vi "MecaKinematics_New.vi"(8 "RearRight":T1 {"Y" format="%14.3f"; "X" format="%14.3f"}, 9 "RearLeft":T1 {"Y" format="%14.3f"; "X" format="%14.3f"}, 10 "FrontRight":T1 {"Y" format="%14.3f"; "X" format="%14.3f"}, 11 "FrontLeft":T1 {"Y" format="%14.3f"; "X" format="%14.3f"}) -> (3 "MECA_DRIVE_KINEMATICS":T2={"FrontLeft"={"X"=0.0, "Y"=0.0}, "FrontRight"={"X"=0.0, "Y"=0.0}, "RearLeft"={"X"=0.0, "Y"=0.0}, "RearRight"={"X"=0.0, "Y"=0.0}, "InverseKinematics"=[[0.0, 1.0, -1.0, 0.0], [0.0, 1.0, 1.0, 0.0], [0.0, 1.0, 1.0, 0.0], [0.0, 1.0, -1.0, 0.0]], "ForwardKinematics"=[[0.0, 1.0, -1.0, 0.0], [0.0, 1.0, 1.0, 0.0], [0.0, 1.0, 1.0, 0.0], [0.0, 1.0, -1.0, 0.0]], "PrevCoR"={"X"=0.0, "Y"=0.0}} {"PrevCoR"."Y" format="%14.3f"; "PrevCoR"."X" format="%14.3f"; "RearRight"."Y" format="%14.3f"; "RearRight"."X" format="%14.3f"; "RearLeft"."Y" format="%14.3f"; "RearLeft"."X" format="%14.3f"; "FrontRight"."Y" format="%14.3f"; "FrontRight"."X" format="%14.3f"; "FrontLeft"."Y" format="%14.3f"; "FrontLeft"."X" format="%14.3f"})   [LabVIEW 2019, in "Trajectory_Library.lvlib"]
doc: "Constructs a MecanumDriveKinematics data structure.\n\nHelper class that converts a chassis velocity (dx, dy, and dtheta components) into individual wheel speeds.\n\nThe inverse kinematics (converting from a desired chassis velocity to individual wheel speeds) uses the relative locations of the wheels with respect to the center of rotation. The center of rotation for inverse kinematics is also variable. This means that you can set your set your center of rotation in a corner of the robot to perform special evasion manuevers.\n \nForward kinematics (converting an array of wheel speeds into the overall chassis motion) is performs the exact opposite of what inverse kinematics does. Since this is an overdetermined system (more equations than variables), we use a least-squares approximation.\n\nThe inverse kinematics: [wheelSpeeds] = [wheelLocations][chassisSpeeds] We take the Moore-Penrose pseudoinverse of [wheelLocations] and then multiply by [wheelSpeeds] to get our chassis speeds.\n \nForward kinematics is also used for odometry -- determining the position of the robot on the field using encoders and a gyro.\n\nParameters:\n - Left Front - The location of the front-left wheel relative to the physical center of the robot. (Translation)\n - Right Front - The location of the front-right wheel relative to the physical center of the robot. (Translation)\n - Left Rear - The location of the rear-left wheel relative to the physical center of the robot. (Translation)\n - Right Rear - The location of the rear-right wheel relative to the physical center of the robot. (Translation)\n\nReturns:\n - Meca_Drive_Kinematics - Data structure"
uses:
  Trajectory_Library.lvlib
  TypeDef/MECA_DRIVE_KINEMATICS.ctl
  TypeDef/TRANSLATION2D.ctl
  <vilib>/Analysis/Matrix/Datatypes/RealMatrix.ctl
  <vilib>/Rock Robotics/SystemInterfaces/NetworkCommunication/NetComm_UsageReport_ResourceType.ctl
  <vilib>/Analysis/_algsub.llb/Real PseudoInverse Matrix.vi
  Util_LibraryGlobals.vi
  <vilib>/Analysis/Matrix/NI_Matrix.lvlib
  <vilib>/Analysis/NI_AALPro.lvlib
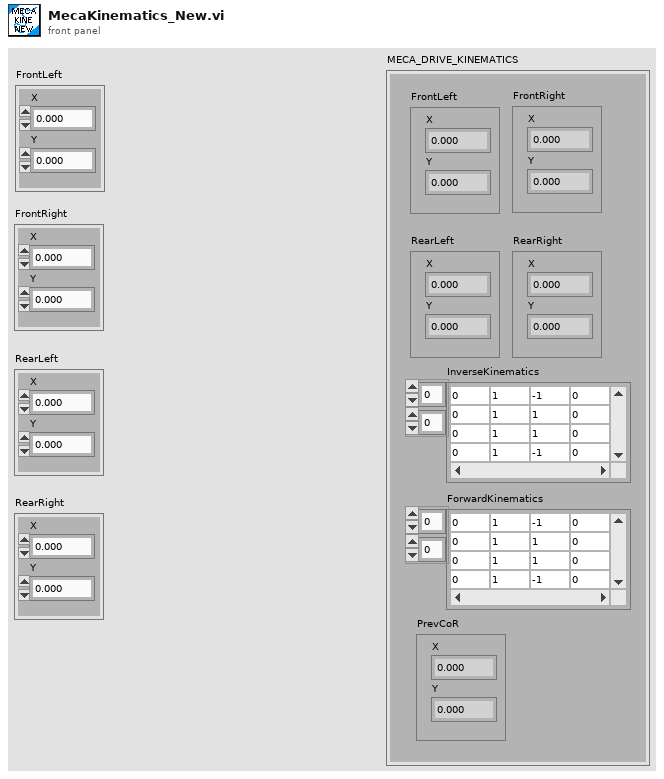
[diagram p1: front panel]
types:
  T1 = typedef "Trajectory_Library.lvlib/TRANSLATION2D.ctl" = cluster{"X":dbl, "Y":dbl}
  T2 = typedef "Trajectory_Library.lvlib/MECA_DRIVE_KINEMATICS.ctl" = cluster{"FrontLeft":T1, "FrontRight":T1, "RearLeft":T1, "RearRight":T1, "InverseKinematics":T3, "ForwardKinematics":T3, "PrevCoR":T1}
  T3 = typedef "NI_Matrix.lvlib/RealMatrix.ctl" = dbl[][]
  T4 = typedef "NetComm_UsageReport_ResourceType.ctl" = enum8{"Controller", "Module", "Language", "CANPlugin", "Accelerometer", "ADXL345", "AnalogChannel", "AnalogTrigger", "AnalogTriggerOutput", "CANJaguar", "Compressor", "Counter", "Dashboard", "DigitalInput", "DigitalOutput", "DriverStationCIO", "DriverStationEIO", "DriverStationLCD", "Encoder", "GearTooth", "Gyro", "I2C", "Framework", "Jaguar", "Joystick", "Kinect", "KinectStick", "PIDController", "Preferences", "PWM", "Relay", "RobotDrive", "SerialPort", "Servo", "Solenoid", "SPI", "Task", "Ultrasonic", "Victor", "Button", "Command", "AxisCamera", "PCVideoServer", "SmartDashboard", "Talon", "HiTechnicColorSensor", "HiTechnicAccel", "HiTechnicCompass", "SRF08", "AnalogOutput", "Victor SP", "Talon SRX", "CAN Talon SRX", "ADXL362 Accel", "ADXRS450 Gyro", "Rev SPARK", "Mindsensors SD540", "Digital Filter", "ADIS16448", "PDP", "PCM", "PigeonIMU", "Nidec Brushless", "CTRE CANifier", "CTRE TalonFX", "CTRE Future 1", "CTRE Future 2", "CTRE Future 3", "CTRE Future 4", "CTRE Future 5", "CTRE Future 6", "Linear Filter", "Xbox Controller", "USB Camera", "NavX", "Pixy", "Pixy2", "ScanseSweep", "Shuffleboard", "CAN", "Digilent DMC60", "PWM Victor SPX", "Rev SPARK MAX PWM", "Rev SPARK MAX CAN", "ADIS16470", "PIDController2", "ProfiledPIDController", "Kinematics", "Odometry", "Units", "Trapezoid Profile", "DutyCycle", "Addressable LEDs", "Fusion Venom"}
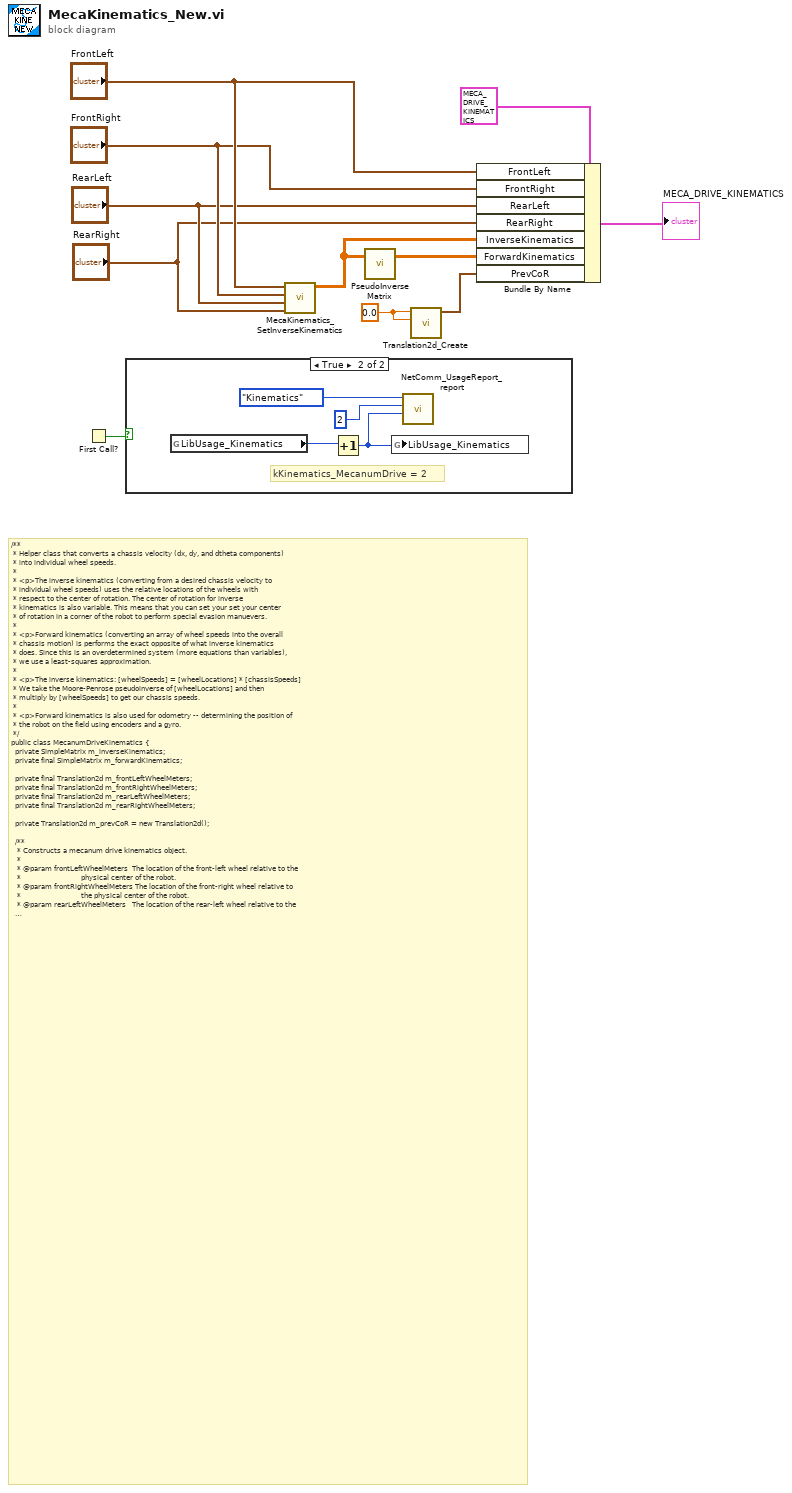
[diagram p0: block diagram]
diagram:
  w2 = 0.0 ("X")
  # "/**\n * Helper class that converts a chassis velocity (dx, dy, and dtheta components)\n * into individual wheel speeds.\n *\n * <p>The inverse kinematics (converting from a desired chassis velocity to\n * individual wheel speeds) uses the relative locations of the wheels with\n * respect to the center of rotation. The center of rotation for inverse\n * kinematics is also variable. This means that you can set your set your center\n * of rotation in a corner of the robot to perform special evasion manuevers.\n *\n * <p>Forward kinematics (converting an array of wheel speeds into the overall\n * chassis motion) is performs the exact opposite of what inverse kinematics\n * does. Since this is an overdetermined system (more equations than variables),\n * we use a least-squares approximation.\n *\n * <p>The inverse kinematics: [wheelSpeeds] = [wheelLocations] * [chassisSpeeds]\n * We take the Moore-Penrose pseudoinverse of [wheelLocations] and then\n * multiply by [wheelSpeeds] to get our chassis speeds.\n *\n * <p>Forward kinematics is also used for odometry -- determining the position of\n * the robot on the field using encoders and a gyro.\n */\npublic class MecanumDriveKinematics {\n  private SimpleMatrix m_inverseKinematics;\n  private final SimpleMatrix m_forwardKinematics;\n\n  private final Translation2d m_frontLeftWheelMeters;\n  private final Translation2d m_frontRightWheelMeters;\n  private final Translation2d m_rearLeftWheelMeters;\n  private final Translation2d m_rearRightWheelMeters;\n\n  private Translation2d m_prevCoR = new Translation2d();\n\n  /**\n   * Constructs a mecanum drive kinematics object.\n   *\n   * @param frontLeftWheelMeters  The location of the front-left wheel relative to the\n   *                              physical center of the robot.\n   * @param frontRightWheelMeters The location of the front-right wheel relative to\n   *                              the physical center of the robot.\n   * @param rearLeftWheelMeters   The location of the rear-left wheel relative to the\n   *                              physical center of the robot.\n   * @param rearRightWheelMeters  The location of the rear-right wheel relative to the\n   *                              physical center of the robot.\n   */\n  public MecanumDriveKinematics(Translation2d frontLeftWheelMeters,\n                                Translation2d frontRightWheelMeters,\n                                Translation2d rearLeftWheelMeters,\n                                Translation2d rearRightWheelMeters) {\n    m_frontLeftWheelMeters = frontLeftWheelMeters;\n    m_frontRightWheelMeters = frontRightWheelMeters;\n    m_rearLeftWheelMeters = rearLeftWheelMeters;\n    m_rearRightWheelMeters = rearRightWheelMeters;\n\n    m_inverseKinematics = new SimpleMatrix(4, 3);\n\n    setInverseKinematics(frontLeftWheelMeters, frontRightWheelMeters,\n        rearLeftWheelMeters, rearRightWheelMeters);\n    m_forwardKinematics = m_inverseKinematics.pseudoInverse();\n\n    HAL.report(tResourceType.kResourceType_Kinematics, tInstances.kKinematics_MecanumDrive);\n  }"
  n1 = First Call?() -> (First Call?: T/F=w1:bool)
  n2 = case shown="True" w1 {
    frame False {
    }
    frame True {
      # "kKinematics_MecanumDrive = 2"
      n3 = global read "Util_LibraryGlobals.vi" "LibUsage_Kinematics"() -> (w14:i32)
      n4 = Increment(x=w14) -> (x+1=w13:i32)
      n5 = global write "Util_LibraryGlobals.vi" "LibUsage_Kinematics"(w13) -> ()
      n6 = call <vilib>:"NetComm_UsageReport_report.vi"("Context"=w13, "Instance Number"=u8 2, "Resource Type"=NetComm_UsageReport_ResourceType."Kinematics") -> ()  [unwired: 9 in]
    }
  }
  n7 = call "MecaKinematics_SetInverseKinematics.vi"("RearRight"="RearRight", "RearLeft"="RearLeft", "FrontRight"="FrontRight", "FrontLeft"="FrontLeft") -> ("InverseKinematics"=w5:T3)  [unwired: 7 in]
  n8 = call-poly <vilib>:"PseudoInverse Matrix.vi"("Input Matrix"=w5) -> ("PseudoInverse Matrix"=w4:T3)  [unwired: 1 in, 1 out]
  n9 = call "Translation2d_Create.vi"("Y"=w2, "X"=w2) -> ("TRANSLATION"=w3:T1)  [unwired: 9 in]
  n10 = Bundle By Name(cluster=T2 {"FrontLeft"={"X"=0.0, "Y"=0.0}, "FrontRight"={"X"=0.0, "Y"=0.0}, "RearLeft"={"X"=0.0, "Y"=0.0}, "RearRight"={"X"=0.0, "Y"=0.0}, "InverseKinematics"=[[0.0, 1.0, -1.0, 0.0], [0.0, 1.0, 1.0, 0.0], [0.0, 1.0, 1.0, 0.0], [0.0, 1.0, -1.0, 0.0]], "ForwardKinematics"=[[0.0, 1.0, -1.0, 0.0], [0.0, 1.0, 1.0, 0.0], [0.0, 1.0, 1.0, 0.0], [0.0, 1.0, -1.0, 0.0]], "PrevCoR"={"X"=0.0, "Y"=0.0}} ("MECA_DRIVE_KINEMATICS"), "FrontLeft"="FrontLeft", "FrontRight"="FrontRight", "RearLeft"="RearLeft", "RearRight"="RearRight", "InverseKinematics"=w5, "ForwardKinematics"=w4, "PrevCoR"=w3) -> (→"MECA_DRIVE_KINEMATICS":T2)
